vi "帮助文档下载.vi"(0 "确定按钮":bool) -> ()   [LabVIEW 2019]
uses:
  <vilib>/Platform/browser.llb/Open URL in Default Browser (path).vi
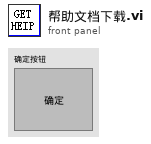
[diagram p1: front panel]
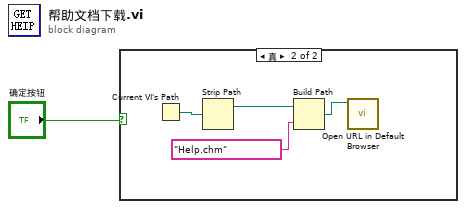
[diagram p0: block diagram]
diagram:
  n1 = case shown="真" "确定按钮" {
    frame False {
    }
    frame True {
      n2 = Current VI's Path() -> (path=w4:path)
      n3 = Strip Path(path=w4) -> (stripped path=w2:path)  [unwired: 1 out]
      n4 = Build Path(base path=w2, name or relative path="Help.chm") -> (appended path=w3:path)
      n5 = call-poly <vilib>:"Open URL in Default Browser.vi"("path"=w3) -> ()  [unwired: 5 in, 2 out]
    }
  }
